vi "Enqueue Data.vi"(8 "error in (no error)":errorcluster, 10 "data":waveform(cdb), 11 "Data Queue in":refnum<queue>) -> (0 "error out":errorcluster)   [LabVIEW 2021]
uses:
  Waveform Queue Data.ctl
  Data Processing.ctl
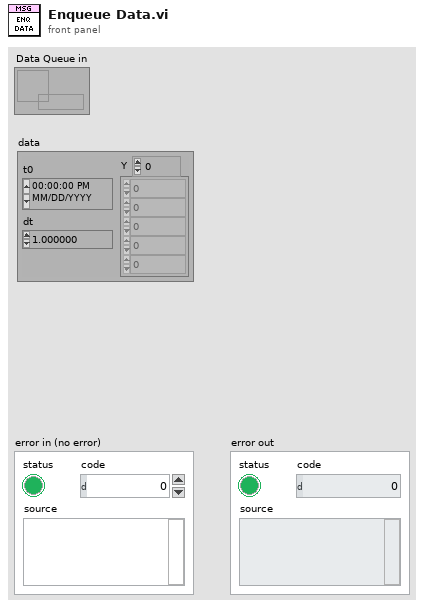
[diagram p1: front panel]
types:
  T1 = typedef "Data Processing.ctl" = enum16{"Initialize TDMS", "Close TDMS", "Write", "Exit"}
  T2 = typedef "Waveform Queue Data.ctl" = cluster{"wfm dat":waveform(cdb), "msg":T1}
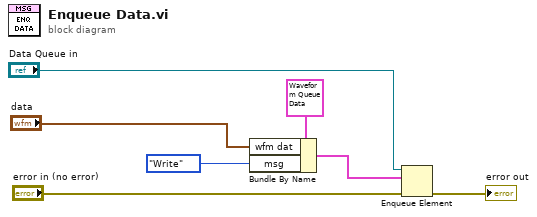
[diagram p0: block diagram]
diagram:
  n1 = Bundle By Name(cluster=T2 {"wfm dat"={"t0"=timestamp(0 s since 1904-01-01), "dt"=0.0, "Y"=[]}, "msg"=enum."Write"} ("element"), "wfm dat"="data", "msg"=Data_Processing."Write") -> (w2:T2)
  n2 = Enqueue Element(queue="Data Queue in", element=w2, error in (no error)="error in (no error)") -> (error out=→"error out":errorcluster)  [unwired: 1 in, 2 out]
